vi "Read Configuration Data.vi"(8 "error in":errorcluster) -> (0 "error out":errorcluster, 3 "MHL Configuration":T1)   [LabVIEW 2021]
uses:
  controls/MHL Configuration.ctl
  <vilib>/Utility/config.llb/NI_LVConfig.lvlib
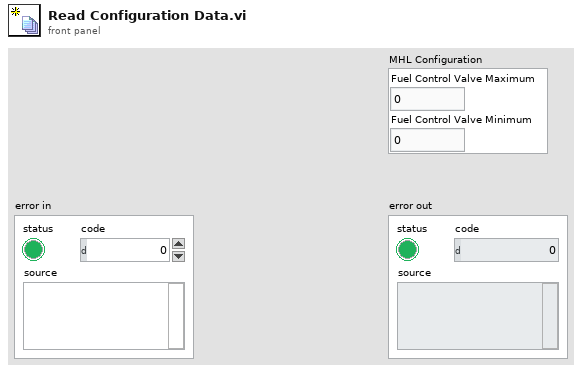
[diagram p1: front panel]
types:
  T1 = typedef "MHL Configuration.ctl" = cluster{"Fuel Control Valve Maximum":dbl, "Fuel Control Valve Minimum":dbl}
  T2 = typedef "NI_LVConfig.lvlib/Config Data RefNum.ctl" = refnum<k1>
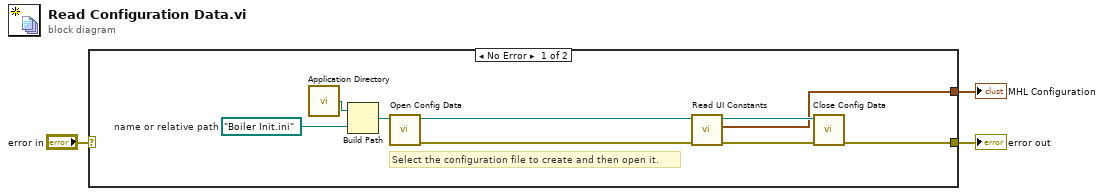
[diagram p0: block diagram]
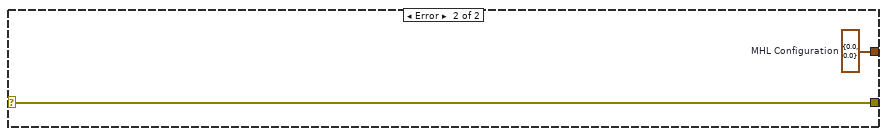
[diagram p2: hidden frame]
diagram:
  n1 = case shown="No Error" "error in" {
    selector: "error in" -> [_ w13]
    tunnel: [w8 w13] -> w2
    tunnel: [w7 w14] -> w1
    frame No Error {
      w4 = path "Boiler Init.ini"  # name or relative path
      # "Select the configuration file to create and then open it."
      n2 = call <vilib>:"Application Directory.vi"() -> ("Application Directory"=w5:path)
      n3 = Build Path(base path=w5, name or relative path=w4) -> (appended path=w6:path)
      n4 = call <vilib>:"Open Config Data.vi"("configuration file path"=w6) -> ("error out"=w12:errorcluster, "refnum"=w11:T2)  [unwired: 8 in, 1 out]
      n5 = call "Read UI Constants.vi"("error in"=w12, "CFG File Refnum in"=w11) -> ("error out"=w10:errorcluster, "MHL Configuration"=w7:T1, "CFG File Refnum out"=w9:T2)  [unwired: 7 in]
      n6 = call <vilib>:"Close Config Data.vi"("error in (no error)"=w10, "refnum"=w9) -> ("error out"=w8:errorcluster)  [unwired: 8 in, 1 out]
    }
    frame Error {
      w14 = T1 {"Fuel Control Valve Maximum"=0.0, "Fuel Control Valve Minimum"=0.0}  # MHL Configuration
    }
  }
  "error out" <- w2
  "MHL Configuration" <- w1
